vi "AMC Dispatch Get All Queues.vi"(8 "error in (no error)":errorcluster, 11 "receiver host":string) -> (0 "error out":errorcluster, 2 "String Response":string)   [LabVIEW 2015]
doc: "This VI is used for compatibility with previous versions of the AMC library. Use the AMC VIs located in the <b>Data Communication >> Asynchronous Message Communication</b> palette."
uses:
  <vilib>/NI/AMC/Message.ctl
  <vilib>/NI/Tools/Keyed Array/KeyedArray.ctl
  <vilib>/NI/AMC/AMC.lvlib
  <vilib>/NI/Tools/Keyed Array/Tools_KeyedArray.lvlib
panel:
  out "Message":T1
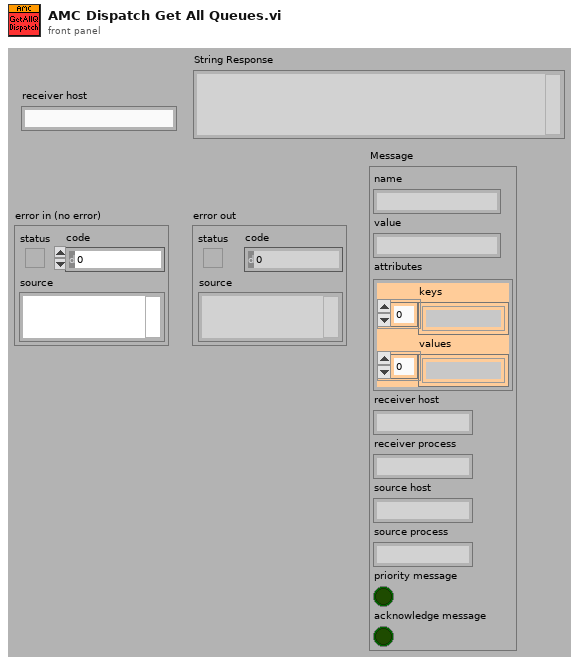
[diagram p1: front panel]
types:
  T1 = typedef "AMC.lvlib/Message.ctl" = cluster{"name":string, "value":string, "attributes":T2, "receiver host":string, "receiver process":string, "source host":string, "source process":string, "priority message":bool, "acknowledge message":bool}
  T2 = typedef "Tools_KeyedArray.lvlib/KeyedArray.ctl" = cluster{"keys":string[], "values":string[]}
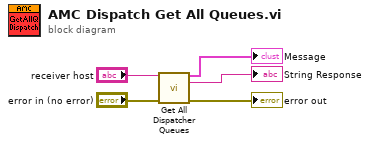
[diagram p0: block diagram]
diagram:
  n1 = call <vilib>:"Get All Dispatcher Queues.vi"("receiver host (\"\")"="receiver host", "error in"="error in (no error)") -> ("response message"=→"Message":T1, "string response"=→"String Response":string, "error out"=→"error out":errorcluster)  [unwired: 10 in, 1 out]
